vi "SSH Async Execute Command.vi"(8 "Error In":errorcluster, 10 "Command":string, 11 "Install LV Data in":T1) -> (0 "Error Out":errorcluster, 3 "Install LV Data out":T1)   [LabVIEW 2020, in "LMH-LINX.lvlib"]
uses:
  LMH-LINX.lvlib
  Target Management/Install LV Data.ctl
  Target Management/Target Info.ctl
  Target Management/NIC Info.ctl
  Target Management/NIC Mode.ctl
  c:/p4/penguin/lvaddon/MakerHub/LINX/trunk/20.1/objects/MakerHub_LINX/win32U/i386/msvc90/release/LabVIEW/vi.lib/MakerHub/LINX/Resources/Renci.SshNet.dll
  Resources/Renci.SshNet.dll
  <vilib>/MakerHub/LINX/Private/Utilties/SSH/SSH Unix Session Op.ctl
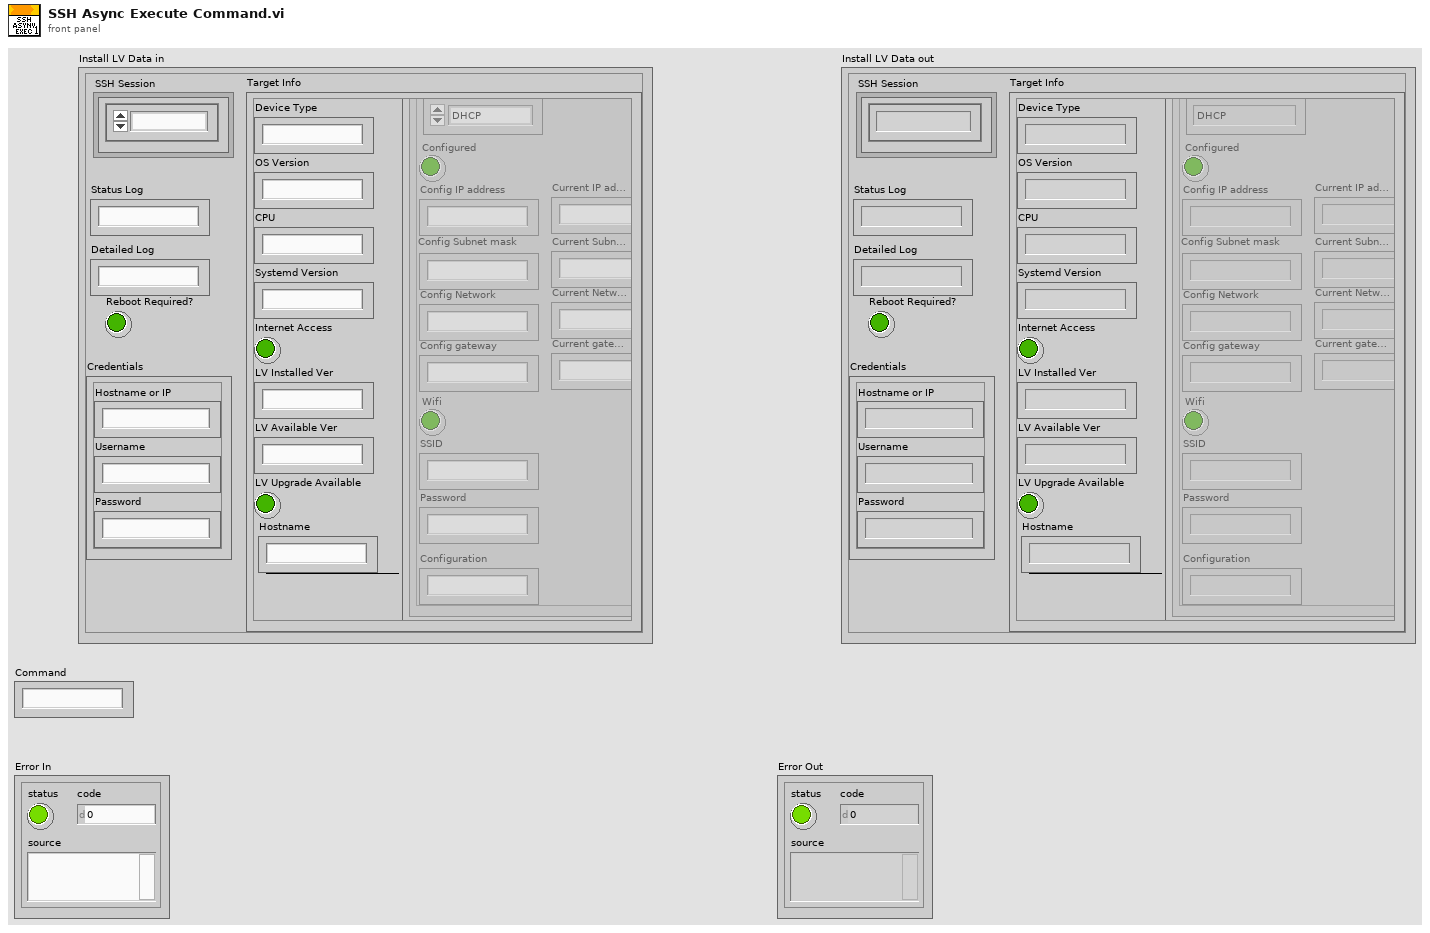
[diagram p1: front panel]
types:
  T1 = typedef "LMH-LINX.lvlib/Install LV Data.ctl" = cluster{"SSH Session":refnum<k1>, "Status Log":string, "Detailed Log":string, "Credentials":cluster{"Hostname or IP":string, "Username":string, "Password":string}, "Target Info":T2, "Reboot Required?":bool}
  T2 = typedef "LMH-LINX.lvlib/Target Info.ctl" = cluster{"OS Version":string, "CPU":string, "Systemd Version":string, "Internet Access":bool, "Device Type":string, "LV Installed Ver":string, "LV Available Ver":string, "LV Upgrade Available":bool, "Hostname":string, "NIC Info":T3[]}
  T3 = typedef "LMH-LINX.lvlib/NIC Info.ctl" = cluster{"Name":string, "NIC Mode":T4, "Configured":bool, "Config IP address":string, "Config Subnet mask":string, "Config Network":string, "Config gateway":string, "Wifi":bool, "SSID":string, "Password":string, "Configuration":string, "Current IP address":string, "Current Subnet mask":string, "Current gateway":string, "Current Network":string}
  T4 = typedef "LMH-LINX.lvlib/NIC Mode.ctl" = enum16{"DHCP", "Static", "Loopback"}
  T5 = typedef "LMH-LINX.lvlib/SSH Unix Session Op.ctl" = enum16{"New", "Get", "Delete"}
  T6 = typedef "LMH-LINX.lvlib/SSH Unix Session Info.ctl" = cluster{"PID":i32, "Read FD":i32, "Write FD":i32, "Error FD":i32}
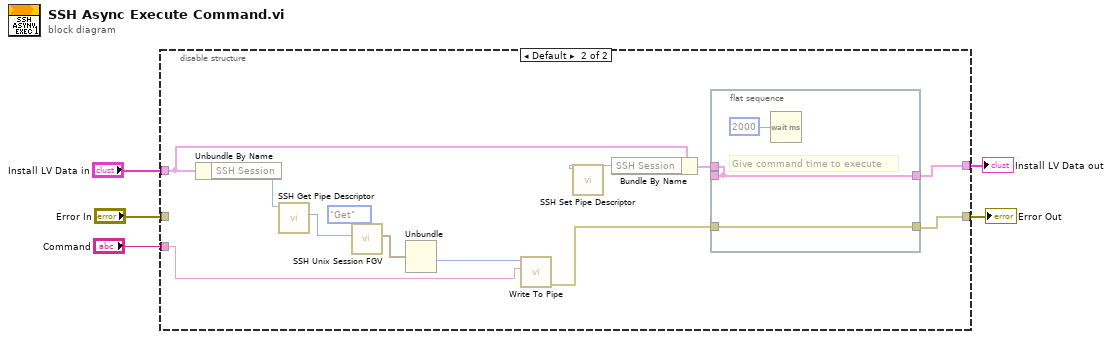
[diagram p0: block diagram]
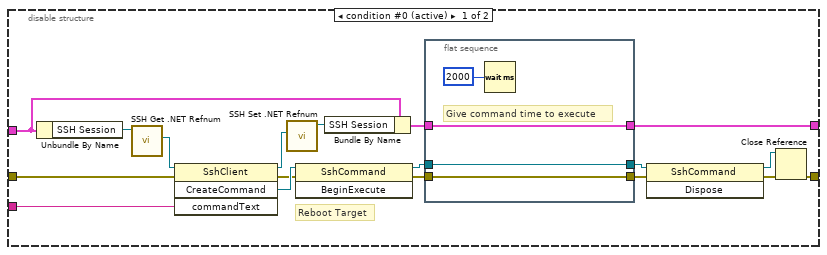
[diagram p2: hidden frame]
diagram:
  n1 = disable-structure shown="Default" {
    disable-tunnel: [w23 w28] -> w5
    disable-tunnel: [w21 w30] -> w4
    disable-tunnel: "Command" -> [w14 w32]
    disable-tunnel: "Error In" -> [w13 _]
    disable-tunnel: "Install LV Data in" -> [w10 w39]
    frame condition #0 (active) {
      # "Reboot Target"
      n2 = Unbundle By Name(w10) -> ("SSH Session"=w9:refnum<k1>)
      n3 = call "SSH Get .NET Refnum.vi"("SSH Session"=w9) -> ("SSH .NET Refnum"=w8:refnum<k24>)  [unwired: 8 in, 2 out]
      n4 = invoke class="SshClient" method="CreateCommand"(reference=w8, error in=w13, "commandText"=w14) -> (reference out=w7:refnum<k24>, error out=w15:errorcluster, "CreateCommand"=w18:refnum<k24>)  [unwired: 1 in, 1 out]
      n5 = call "SSH Set .NET Refnum.vi"("SSH .NET Refnum"=w7) -> ("SSH Session"=w6:refnum<k1>)  [unwired: 9 in, 1 out]
      n6 = invoke class="SshCommand" method="BeginExecute"(reference=w18, error in=w15) -> (reference out=w20:refnum<k24>, error out=w17:errorcluster)  [unwired: 1 in, 1 out]
      n7 = Bundle By Name(cluster=w10, "SSH Session"=w6) -> (w22:T1)
      n8 = flat-sequence {
        tunnel: [w26] -> w16
        tunnel: w17 -> [w26]
        tunnel: [w25] -> w19
        tunnel: w20 -> [w25]
        tunnel: [w24] -> w21
        tunnel: w22 -> [w24]
        frame #0 {
          # "Give command time to execute"
          n9 = Wait (ms)(milliseconds to wait=u32 2000) -> ()  [unwired: 1 out]
        }
      }
      n10 = invoke class="SshCommand" method="Dispose"(reference=w19, error in=w16) -> (reference out=w12:refnum<k24>, error out=w11:errorcluster)  [unwired: 1 in, 1 out]
      n11 = Close Reference(reference=w12, error in (no error)=w11) -> (error out=w23:errorcluster)
    }
    frame condition #1 {
      n12 = Unbundle By Name(w39) -> ("SSH Session"=w38:refnum<k1>)
      n13 = call <vilib>:"SSH Get Pipe Descriptor.vi"("SSH Session"=w38) -> ("SSH Pipe Descriptor"=w33:i32)  [unwired: 8 in, 2 out]
      n14 = call <vilib>:"SSH Unix Session FGV.vi"("Session In"=w33, "Operation"=SSH_Unix_Session_Op."Get") -> ("info in"=w35:T6)  [unwired: 8 in, 1 out]
      n15 = Unbundle(w35) -> ("Write FD"=w34:i32)  [unwired: 3 out]
      n16 = call <vilib>:"Write To Pipe.vi"("data"=w32, "file descriptor"=w34) -> ("error out"=w29:errorcluster)  [unwired: 3 in, 2 out]
      n17 = call <vilib>:"SSH Set Pipe Descriptor.vi"() -> ("SSH Session"=w37:refnum<k1>)  [unwired: 10 in, 1 out]
      n18 = Bundle By Name(cluster=w39, "SSH Session"=w37) -> (w31:T1)
      n19 = flat-sequence {
        tunnel: [w41] -> w28
        tunnel: w29 -> [w41]
        tunnel: [w40] -> w30
        tunnel: [w40] -> _
        tunnel: w31 -> [w40]
        frame #0 {
          # "Give command time to execute"
          n20 = Wait (ms)(milliseconds to wait=u32 2000) -> ()  [unwired: 1 out]
        }
      }
    }
  }
  "Error Out" <- w5
  "Install LV Data out" <- w4
